vi "Measure Multiple Times.vi"(0 "Register Buses":refnum<class "ni579x Register Bus v1 Host.lvclass">[](array[class]), 5 "Number of measurements":u16=1000, 11 "error in":errorcluster, 12 "sync.cptr.period":u16, 13 "sync.meas.oversample factor":u16[](array[numeric])) -> (4 "Register Buses (out)":refnum<class "ni579x Register Bus v1 Host.lvclass">[](array[class]), 6 "mode relative offsets":u16[](array[numeric]), 15 "error out":errorcluster)   [LabVIEW 2012, in "ni579x Synchronization v1 Host.lvlib"]
uses:
  <instrlib>/ni579x/Synchronization/v1/Host/ni579x Synchronization v1 Host.lvlib
  <instrlib>/ni579x/Register Bus/v1/Host/ni579x Register Bus v1 Host.lvclass
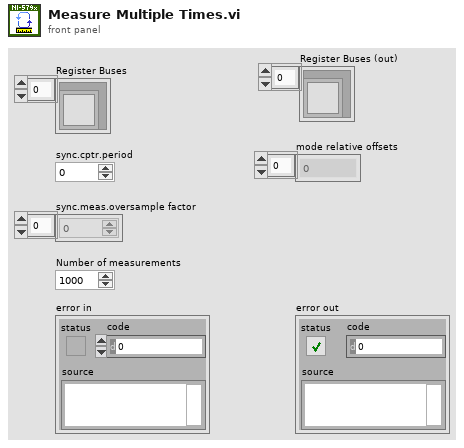
[diagram p1: front panel]
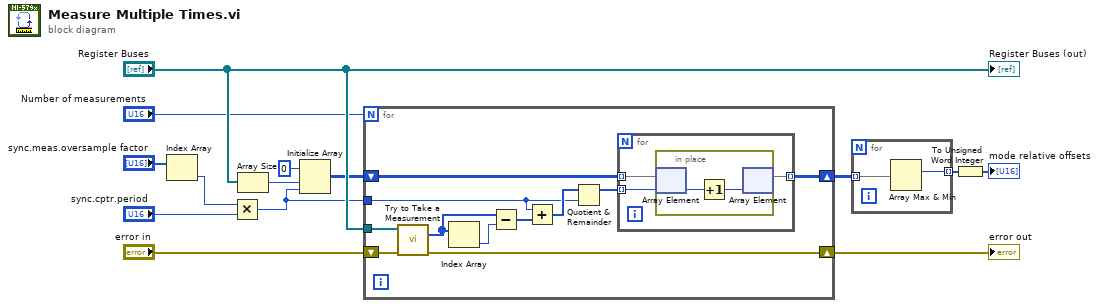
[diagram p0: block diagram]
diagram:
  n1 = Index Array(array="sync.meas.oversample factor") -> (element=w2:u16)  [unwired: 1 in]
  n2 = Multiply(x=w2, y="sync.cptr.period") -> (x*y=w1:u16)
  n3 = Array Size(array="Register Buses") -> (size(s)=w10:i32)
  n4 = Initialize Array(u16 0 ("element"), w10, w1) -> (w9:u16[][])
  n5 = for {
    N: "Number of measurements" -> [_]
    tunnel: "Register Buses" -> [w21]
    shift-right: [w23] -> w5
    shift-left: "error in" -> [w22]
    shift-right: [w24] -> w11
    shift-left: w9 -> [w25]
    tunnel: w1 -> [w16]
    n6 = call <instrlib>:"Try to Take a Measurement.vi"("Register Buses"=w21, "error in"=w22) -> ("measurement values"=w19:u16[], "error out"=w23:errorcluster)  [unwired: 11 in, 1 out]
    n7 = Index Array(array=w19) -> (element=w20:u16)  [unwired: 1 in]
    n8 = Subtract(x=w19, y=w20) -> (x-y=w18:u16[])
    n9 = Add(x=w16, y=w18) -> (x+y=w17:u16[])
    n10 = Quotient & Remainder(x=w17, y=w16) -> (x-y*floor(x/y)=w15:u16[])  [unwired: 1 out]
    n11 = for {
      tunnel: w15 -> [w27] mode=indexing
      tunnel: w25 -> [w28] mode=indexing
      tunnel: [w26] -> w24 mode=indexing
      n12 = in-place {
        n13 = in-place-array #1(w28, w27) -> (w30:u16)
        n14 = Increment(x=w30) -> (x+1=w29:u16)
        n15 = in-place-array #1(w29) -> (w26:u16[])  [unwired: 1 out]
      }
    }
  }
  "error out" <- w5
  n16 = for {
    tunnel: w11 -> [w32] mode=indexing
    tunnel: [w31] -> w14 mode=indexing
    n17 = Array Max & Min(array=w32) -> (max index (indices)=w31:i32)  [unwired: 3 out]
  }
  n18 = To Unsigned Word Integer(number=w14) -> (unsigned 16bit integer=→"mode relative offsets":u16[])
  "Register Buses (out)" <- "Register Buses"
